vi "Interference 1065-366 Textfile.vi"() -> (3 "Tabelle für Textdatei":string[](array[string]))   [LabVIEW 2020, in "EPA 1065.lvlib" / "Interference verificaton 1065-366.lvlib"]
uses:
  Interference verificaton 1065-366.lvlib
  Visualisierungs Elemente/String - Ausgabefeld.ctl
  Ergebnis.ctl
  Sprachverwaltung/FGV Aktion Tabelle zerlegen.ctl
  Aktion FGV Interference.ctl
  Seiten/FT-IR/FGV FT-IR Aktionen.ctl
  Aktion Index uebersetzten.ctl
  Seiten/System Einstellungen V2/Aktioen FGV System Konstanten.ctl
  Sprachverwaltung/Sprachverwaltung.lvlib
  Seiten/System Einstellungen V2/System Einstellungen V2.lvlib
  Seiten/FT-IR/FT-IR.lvlib
panel:
  out "Tabellen-String":string
  out "Ergebnis":T1
  out "error out":errorcluster caption="Fehler (Ausgang)"
  in  "error in (no error)":errorcluster caption="Fehler (Eingang, kein Fehler)"
  out "max. Flow Weighted Mean:":T2 caption="%"
  out "Konzentration FlowWeightedMean":sgl=120.0 caption="Concentration:" min=0 format="%#.2f"
  out "Konzentration Komponente":sgl=120.0 caption="Concentration:" min=0
  out "Komponente:":T2 caption="ppm"
  out "[%]":sgl=120.0 caption="Interference:" min=0 format="%#.6g"
  out "Grenze in ppm:":sgl=2.0 min=0 format="%#.6g"
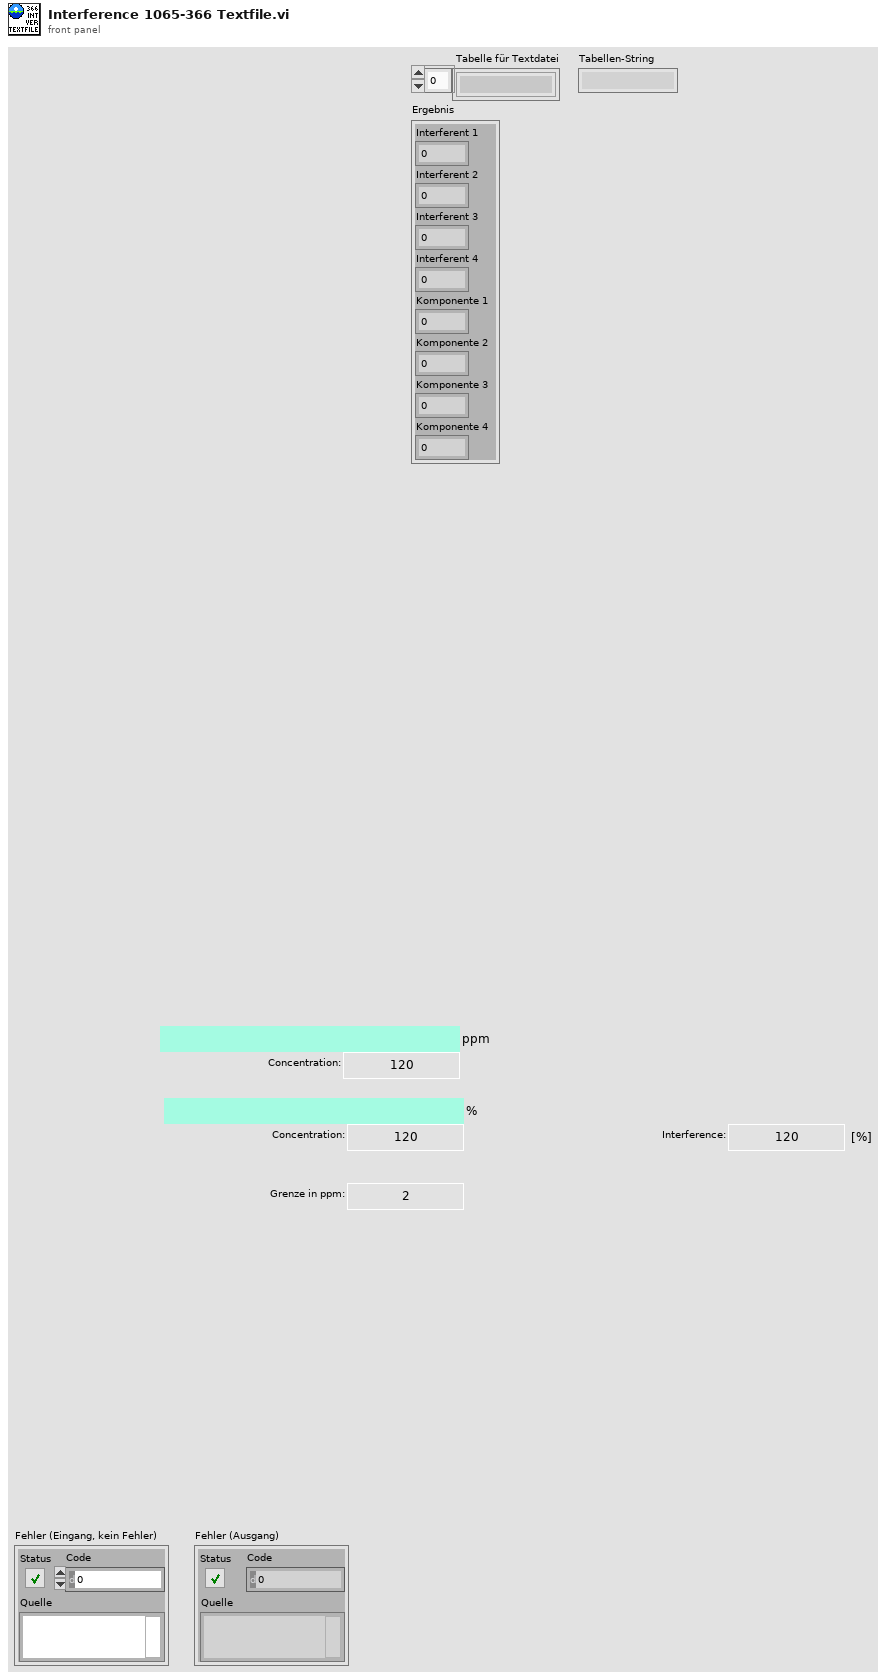
[diagram p1: front panel]
types:
  T1 = typedef "EPA 1065.lvlib/Interference verificaton 1065-366.lvlib/Ergebnis.ctl" = cluster{"Interferent 1":sgl, "Interferent 2":sgl, "Interferent 3":sgl, "Interferent 4":sgl, "Komponente 1":sgl, "Komponente 2":sgl, "Komponente 3":sgl, "Komponente 4":sgl}
  T2 = typedef "String - Ausgabefeld.ctl" = string
  T3 = typedef "System Einstellungen V2.lvlib/Aktioen FGV System Konstanten.ctl" = enum16{"lesen", "laden", "speichern", "Sprache"}
  T4 = typedef "EPA 1065.lvlib/Interference verificaton 1065-366.lvlib/Aktion Index uebersetzten.ctl" = enum16{"lesen", "schreiben", "auswerten"}
  T5 = typedef "FT-IR.lvlib/FGV FT-IR Aktionen.ctl" = enum16{"lesen", "NOG setzen", "NOS setzen", "Initialisieren", "speichern", "ALLES setzen", "FT-IR Spektrum loggen", "Komm Stoppen", "Spektrum LogKonfig"}
  T6 = typedef "EPA 1065.lvlib/Interference verificaton 1065-366.lvlib/Aktion FGV Interference.ctl" = enum16{"Lesen", "TestKonfig", "TestSetting", "Einheiten", "Ergebnis", "Laden", "Tabelle", "Speichern", "löschen"}
  T7 = typedef "Sprachverwaltung.lvlib/FGV Aktion Tabelle zerlegen.ctl" = enum16{"laden", "vereinzeln", "speichern"}
  T8 = typedef "EPA 1065.lvlib/Interference verificaton 1065-366.lvlib/TestSetting.ctl" = cluster{"Bearbeiter:":string, "Pfad:":path, "Textname:":string, "Analysator":T9}
  T9 = typedef "System Einstellungen V2.lvlib/Analysatoren.ctl" = string
  T10 = typedef "EPA 1065.lvlib/Interference verificaton 1065-366.lvlib/TestKonfig.ctl" = cluster{"CH4:":u16, "Ethane:":u16, "NMHC:":u16, "NMNEHC:":u16, "Komp 1 aktiv:":bool, "Komp 2 aktiv:":bool, "Komp 3 aktiv:":bool, "Komp 4 aktiv:":bool, "Modus":T11, "CG Aufschaltzeit:":dbl, "Interferent 1: CO2":u16, "Interferent 2: H2O":u16, "Interferent 3: CH4":u16, "Interferent 4: C2H6 / C3H8":u16, "Gasflaschen Nr.:":string, "Gasflaschen Nr.: 3":string, "Gasflaschen Nr.: 4":string, "Inter 1 aktiv":bool, "Inter 2 aktiv":bool, "Inter 3 aktiv":bool, "Inter 4 aktiv":bool, "Accuracy":string, "Accuracy 3":string, "Accuracy 4":string, "Konzentration 1:":dbl, "Konzentration 2:":dbl, "Konzentration 3:":dbl, "Konzentration 4:":dbl, "Flow weighted mean 1:":dbl, "Flow weighted mean 2:":dbl, "Flow weighted mean 3:":dbl, "Flow weighted mean 4:":dbl}
  T11 = typedef "EPA 1065.lvlib/Interference verificaton 1065-366.lvlib/Modus.ctl" = u16
  T12 = typedef "EPA 1065.lvlib/Interference verificaton 1065-366.lvlib/Komponenten.ctl" = cluster{"Komponente":T2, "Komponente Index":i32, "Komponente 2":T2, "Komponente Index 2":i32, "Komponente 3":T2, "Komponente Index 3":i32, "Komponente 4":T2, "Komponente Index 4":i32, "Interferent 1":T2, "Interferent Index":i32, "Interferent 2":T2, "Interferent 2 Index":i32, "Interferent 3":T2, "Interferent 3 Index":i32, "Interferent 4":T2, "Interferent 4 Index":i32}
  T13 = cluster{"Modell":string, "ProjektNummer":string, "Software Version":string, "Seriennummer":string}
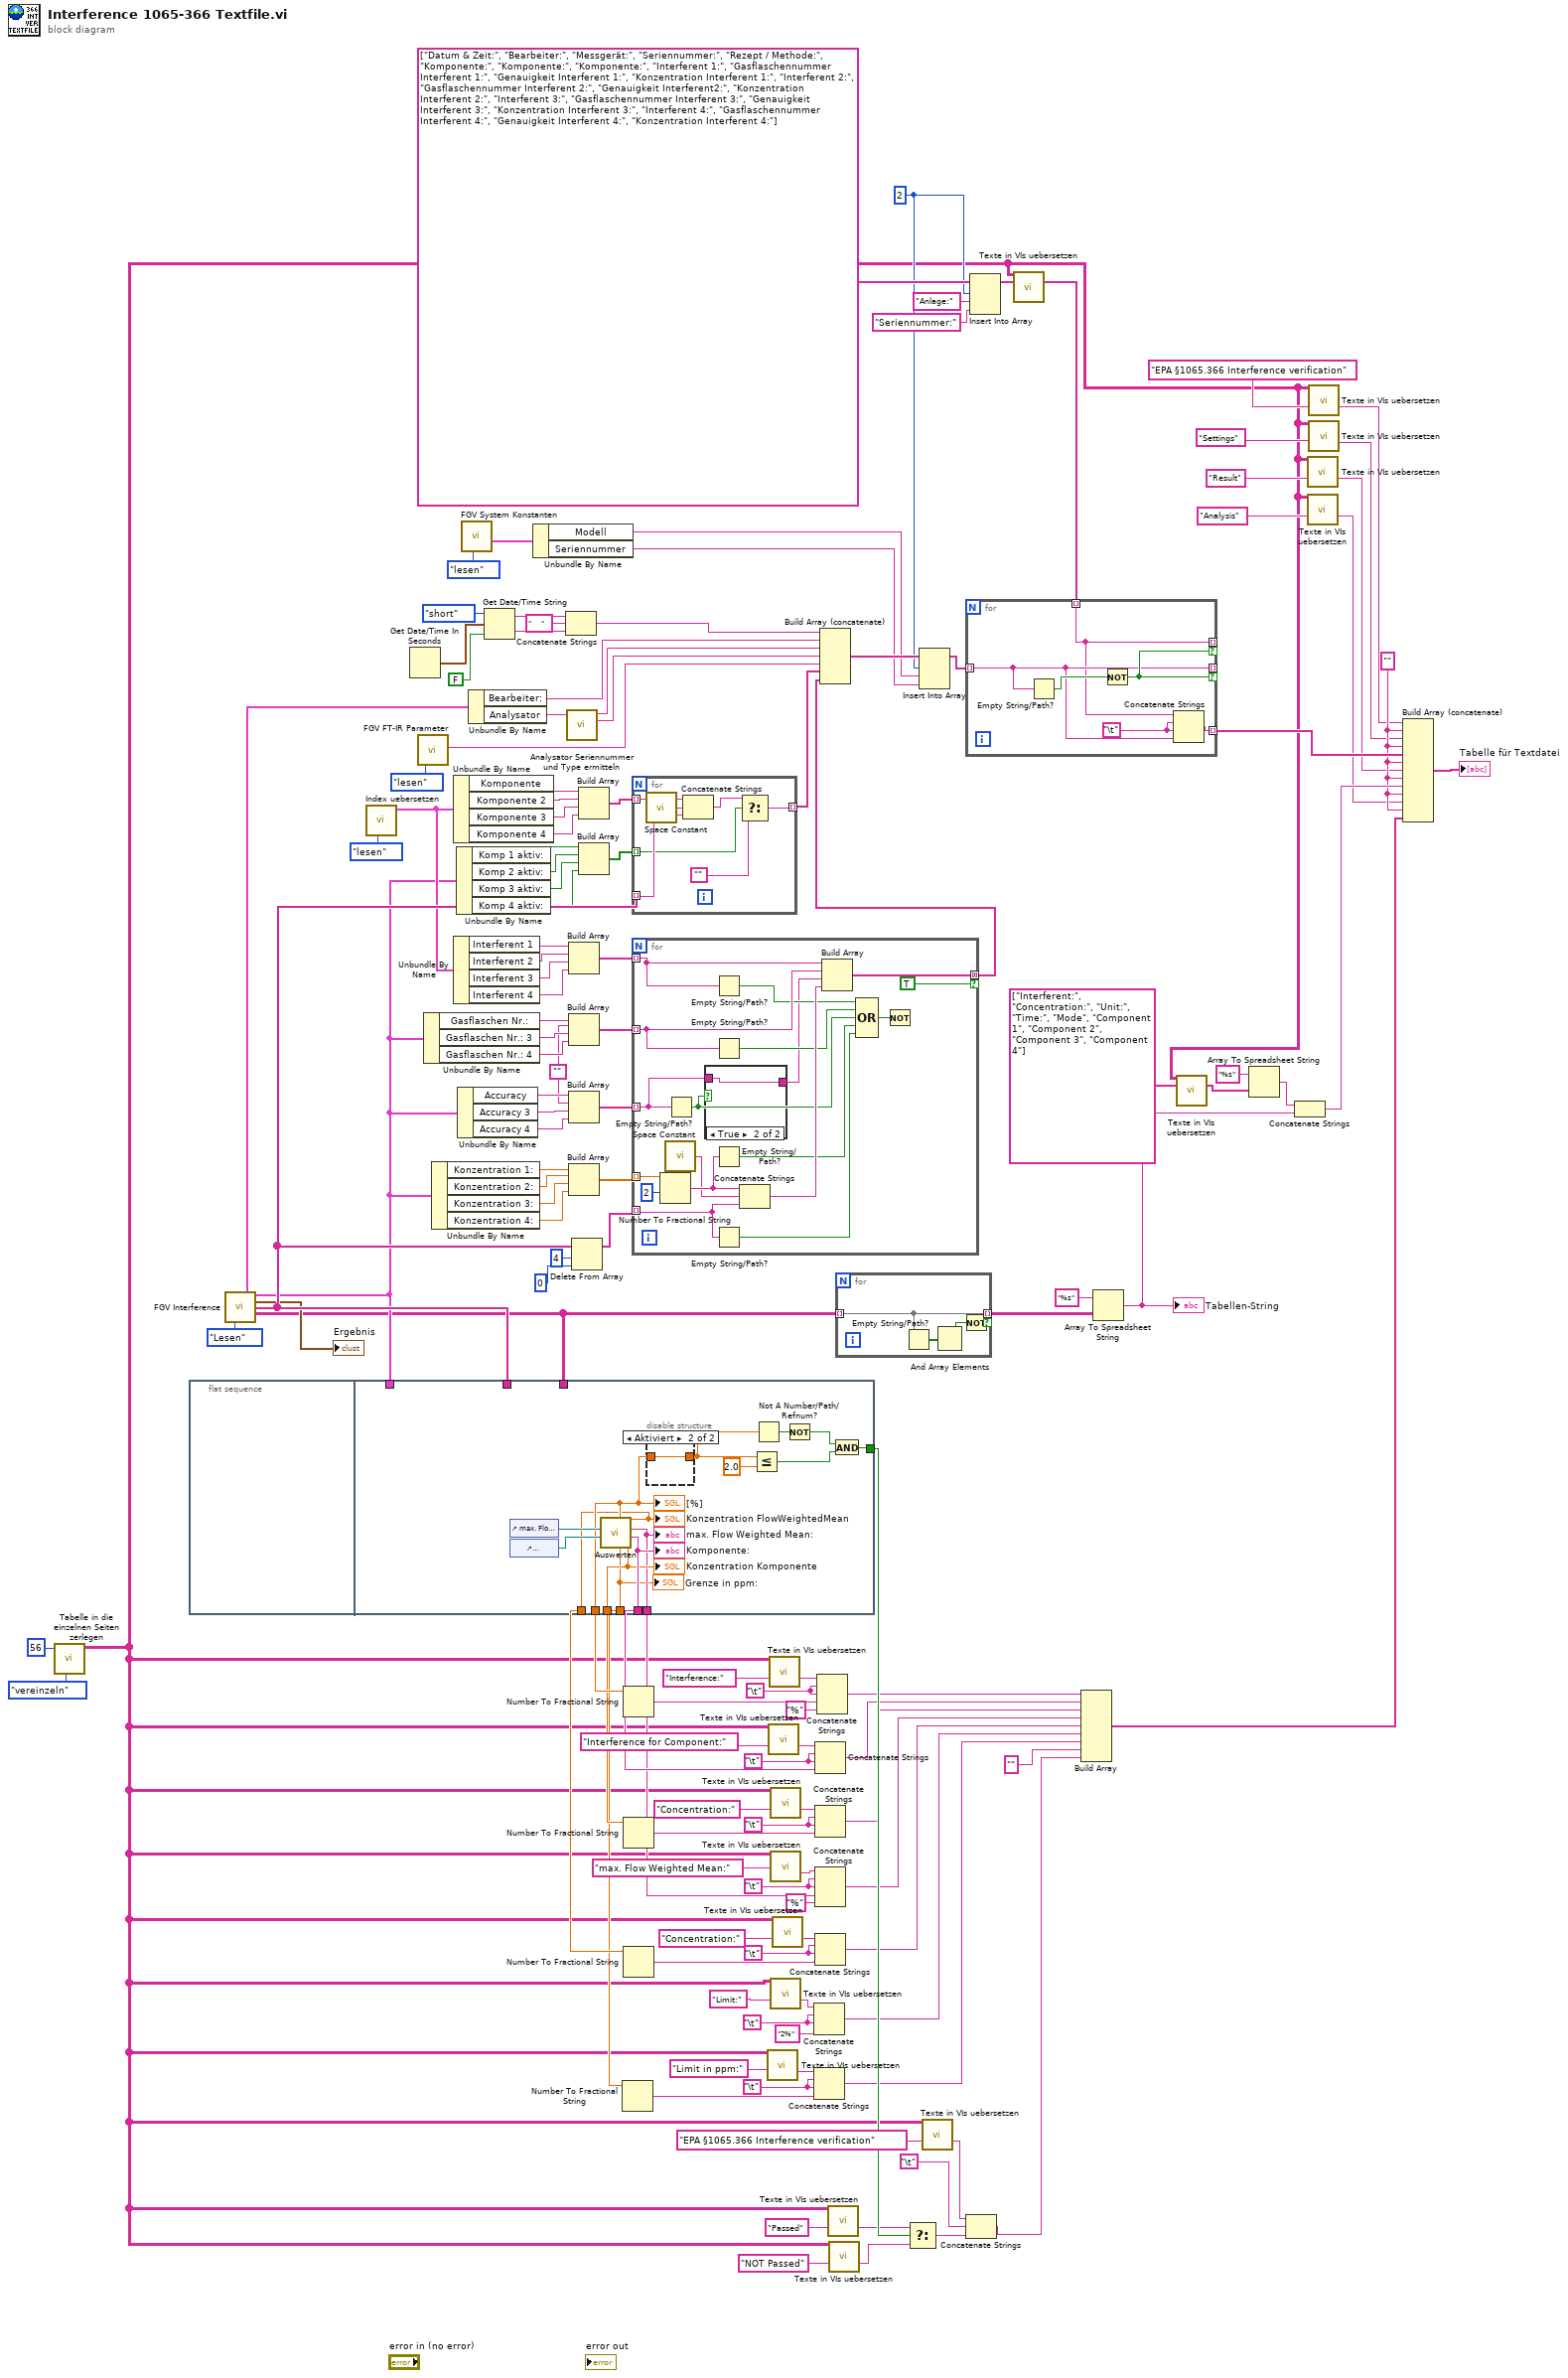
[diagram p0: block diagram]
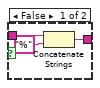
[diagram p2: hidden frame]
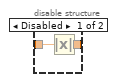
[diagram p3: hidden frame]
diagram:
  w40 = "" ("Element")
  w53 = "\t"
  w54 = "\t"
  w55 = "\t"
  w56 = "\t"
  w57 = "\t"
  w58 = "\t"
  w59 = "\t"
  w81 = ""
  w82 = 2 ("Index")
  n1 = call "Tabelle in die einzelnen Seiten zerlegen.vi"("Aktion"=FGV_Aktion_Tabelle_zerlegen."vereinzeln", "Index (Seite)"=56) -> ("Sprachliste"=w4:string[][])  [unwired: 7 in, 2 out]
  n2 = flat-sequence {
    tunnel: [w149] -> w140
    tunnel: w117 -> [_]
    tunnel: w45 -> [_]
    tunnel: w48 -> [_]
    tunnel: [w148] -> w79
    tunnel: [w147] -> w76
    tunnel: [w146] -> w72
    tunnel: [w145] -> w71
    tunnel: [w144] -> w66
    tunnel: [w143] -> w64
    frame #0 {
    }
    frame #1 {
      n3 = control-ref of="max. Flow Weighted Mean:"() -> (w156:refnum<vi>)
      n4 = control-ref of="Komponente:"() -> (w155:refnum<vi>)
      n5 = call "Auswerten.vi"("Komponente:"=w155, "max. Flow Weighted Mean:"=w156) -> ("Konzentration Komponente"=w146:dbl, "Komponente:"=w147:T2, "max. Flow Weighted Mean:"=w145:T2, "Konzentration FlowWeightedMean"=w144:dbl, "Limit in ppm"=w143:dbl, "[%]"=w148:dbl)  [unwired: 4 in]
      "max. Flow Weighted Mean:" <- w145
      "Konzentration FlowWeightedMean" <- w144
      "Konzentration Komponente" <- w146
      "Komponente:" <- w147
      "[%]" <- w148
      "Grenze in ppm:" <- w143
      n6 = disable-structure shown="Aktiviert" {
        disable-tunnel: [w158 w159] -> w153
        disable-tunnel: w148 -> [w157 w159]
        frame Disabled {
          n7 = Absolute Value(x=w157) -> (abs(x)=w158:dbl)
        }
        frame Enabled {
        }
      }
      n8 = Less Or Equal?(x=w153, y=2.0) -> (x <= y?=w151:bool)
      n9 = Not A Number/Path/Refnum?(number/path/refnum=w153) -> (NaN/Path/Refnum?=w152:bool)
      n10 = Not(x=w152) -> (.not. x?=w150:bool)
      n11 = And(x=w150, y=w151) -> (x .and. y?=w149:bool)
    }
  }
  n12 = call "FGV Interference.vi"("Aktion FGV Interference"=Aktion_FGV_Interference."Lesen") -> ("TestSetting"=w138:T8, "TestKonfig"=w48:T10, "Ergebnis"=→"Ergebnis":T1, "Êinheiten"=w117:string[], "Tabelle"=w45:T2[][])  [unwired: 9 in, 1 out]
  n13 = call "Index uebersetzen.vi"("Aktion"=Aktion_Index_uebersetzten."lesen") -> ("Komponenten"=w111:T12)  [unwired: 9 in, 1 out]
  n14 = Get Date/Time In Seconds() -> (seconds since 1Jan1904=w137:timestamp)
  n15 = call "FGV FT-IR Parameter.vi"("Aktion"=FGV_FT-IR_Aktionen."lesen") -> ("Current Recipe"=w118:string)  [unwired: 11 in, 7 out]
  n16 = Unbundle By Name(w48) -> ("Gasflaschen Nr.:"=w110:string, "Gasflaschen Nr.: 3"=w109:string, "Gasflaschen Nr.: 4"=w108:string)
  n17 = Unbundle By Name(w48) -> ("Konzentration 1:"=w107:dbl, "Konzentration 2:"=w106:dbl, "Konzentration 3:"=w105:dbl, "Konzentration 4:"=w104:dbl)
  n18 = Unbundle By Name(w111) -> ("Komponente"=w129:T2, "Komponente 2"=w128:T2, "Komponente 3"=w127:T2, "Komponente 4"=w38:T2)
  n19 = Unbundle By Name(w111) -> ("Interferent 1"=w115:T2, "Interferent 2"=w114:T2, "Interferent 3"=w113:T2, "Interferent 4"=w112:T2)
  n20 = Unbundle By Name(w48) -> ("Komp 1 aktiv:"=w126:bool, "Komp 2 aktiv:"=w125:bool, "Komp 3 aktiv:"=w124:bool, "Komp 4 aktiv:"=w37:bool)
  n21 = Unbundle By Name(w48) -> ("Accuracy"=w97:string, "Accuracy 3"=w96:string, "Accuracy 4"=w95:string)
  n22 = call "FGV System Konstanten.vi"("Aktionen"=Aktioen_FGV_System_Konstanten."lesen") -> ("Cluster out"=w90:T13)  [unwired: 6 in, 4 out]
  n23 = Unbundle By Name(w138) -> ("Bearbeiter:"=w120:string, "Analysator"=w3:T9)
  n24 = Get Date/Time String(date format (0)=enum16{"short", "long", "abbreviated"}."short" ("Datumsformat (0)"), seconds (now)=w137, want seconds? (F)=FALSE ("Angabe von Sekunden? (F)")) -> (date string=w136:string, time string=w135:string)
  n25 = Unbundle By Name(w90) -> ("Modell"=w86:string, "Seriennummer"=w85:string)
  n26 = Concatenate Strings(w136, "     " ("String"), w135) -> (w121:string)
  n27 = call "Analysator Seriennummer und Type ermitteln.vi"("Analysator"=w3) -> ("Type"=w2:string, "Name für Protokoll"=w1:string)  [unwired: 8 in, 1 out]
  n28 = Build Array(w115, w114, w113, w112) -> (w103:T2[])
  n29 = Build Array(w110, w81, w109, w108) -> (w102:string[])
  n30 = Build Array(w97, w81, w96, w95) -> (w94:string[])
  n31 = Build Array(w107, w106, w105, w104) -> (w101:dbl[])
  n32 = Delete From Array(array=w117, length=4 ("Länge"), index=0 ("Index")) -> (array with subset deleted=w99:string[])  [unwired: 1 out]
  n33 = Build Array(w129, w128, w127, w38) -> (w123:T2[])
  n34 = Build Array(w126, w125, w124, w37) -> (w122:bool[])
  n35 = Number To Fractional String(number=w64) -> (F-format string=w65:string)  [unwired: 3 in]
  n36 = Number To Fractional String(number=w79) -> (F-format string=w80:string)  [unwired: 3 in]
  n37 = Number To Fractional String(number=w72) -> (F-format string=w73:string)  [unwired: 3 in]
  n38 = Number To Fractional String(number=w66) -> (F-format string=w67:string)  [unwired: 3 in]
  n39 = for {
    tunnel: [w163] -> w119 mode=indexing
    tunnel: w123 -> [w166] mode=indexing
    tunnel: w122 -> [w162] mode=indexing
    tunnel: w117 -> [w165] mode=indexing
    n40 = call <vilib>:"Space Constant.vi"() -> ("String"=w164:string)
    n41 = Concatenate Strings(w166, w164, w165) -> (w161:string)
    n42 = Select(t=w161, s=w162, f="") -> (s? t:f=w163:string)
  }
  n43 = for {
    tunnel: w103 -> [w181] mode=indexing
    tunnel: w102 -> [w180] mode=indexing
    tunnel: w101 -> [w184] mode=indexing
    tunnel: w99 -> [w183] mode=indexing
    tunnel: [w178] -> w98 mode=concatenating if=TRUE
    tunnel: w94 -> [w168] mode=indexing
    n44 = Number To Fractional String(number=w184, precision (6)=i16 2 ("Genauigkeit (6)")) -> (F-format string=w182:string)  [unwired: 2 in]
    n45 = call <vilib>:"Space Constant.vi"() -> ("String"=w172:string)
    n46 = Empty String/Path?(string/path=w168) -> (empty?=w167:bool)
    n47 = case shown="True" w167 {
      tunnel: [w186 w188] -> w171
      tunnel: w168 -> [w185 w188]
      frame False {
        n48 = Concatenate Strings(w185, "%" ("String")) -> (w186:string)
      }
      frame True {
      }
    }
    n49 = Empty String/Path?(string/path=w181) -> (empty?=w177:bool)
    n50 = Empty String/Path?(string/path=w180) -> (empty?=w176:bool)
    n51 = Empty String/Path?(string/path=w182) -> (empty?=w173:bool)
    n52 = Empty String/Path?(string/path=w183) -> (empty?=w175:bool)
    n53 = Concatenate Strings(w182, w172, w183) -> (w179:string)
    n54 = Build Array(w181, w180, w171, w179) -> (w178:T2[])
    n55 = Compound Arithmetic op=OR ("Mehrfacharithmetik")(w177, w176, w167, w173, w175) -> (w174:bool)
    n56 = Not(x=w174) -> ()  [unwired: 1 out]
  }
  n57 = call "Texte in VIs uebersetzen.vi"("Sprachliste"=w4, "String zum Übersetzen"="Limit in ppm:" ("String")) -> ("String zum Übersetzen"=w13:string)  [unwired: 9 in, 4 out]
  n58 = call "Texte in VIs uebersetzen.vi"("Sprachliste"=w4, "String zum Übersetzen"="Interference for Component:" ("String")) -> ("String zum Übersetzen"=w23:string)  [unwired: 9 in, 4 out]
  n59 = call "Texte in VIs uebersetzen.vi"("Sprachliste"=w4, "String zum Übersetzen"="Interference:" ("String")) -> ("String zum Übersetzen"=w25:string)  [unwired: 9 in, 4 out]
  n60 = call "Texte in VIs uebersetzen.vi"("Sprachliste"=w4, "String zum Übersetzen"="Concentration:" ("String")) -> ("String zum Übersetzen"=w22:string)  [unwired: 9 in, 4 out]
  n61 = call "Texte in VIs uebersetzen.vi"("Sprachliste"=w4, "String zum Übersetzen"="max. Flow Weighted Mean:" ("String")) -> ("String zum Übersetzen"=w20:string)  [unwired: 9 in, 4 out]
  n62 = call "Texte in VIs uebersetzen.vi"("Sprachliste"=w4, "String zum Übersetzen"="Limit:" ("String")) -> ("String zum Übersetzen"=w16:string)  [unwired: 9 in, 4 out]
  n63 = call "Texte in VIs uebersetzen.vi"("Sprachliste"=w4, "String zum Übersetzen"="Concentration:" ("String")) -> ("String zum Übersetzen"=w18:string)  [unwired: 9 in, 4 out]
  n64 = Concatenate Strings(w16, w53, w53, "2%" ("String")) -> (w51:string)
  n65 = Concatenate Strings(w13, w54, w54, w65) -> (w52:string)
  n66 = Concatenate Strings(w23, w58, w58, w76) -> (w75:string)
  n67 = Concatenate Strings(w22, w57, w57, w73) -> (w74:string)
  n68 = Concatenate Strings(w20, w56, w56, w71, T2 "%" ("String")) -> (w70:string)
  n69 = Concatenate Strings(w18, w55, w55, w67) -> (w68:string)
  n70 = Concatenate Strings(w25, w59, w59, w80, "%" ("String")) -> (w77:string)
  n71 = Build Array (concatenate)(w121, w120, w1, w2, w118, w119, w98) -> (w88:T2[])
  n72 = call "Texte in VIs uebersetzen.vi"("Sprachliste"=w4, "String zum Übersetzen"=T2 "Passed" ("String")) -> ("String zum Übersetzen"=w9:string)  [unwired: 9 in, 4 out]
  n73 = call "Texte in VIs uebersetzen.vi"("Sprachliste"=w4, "String zum Übersetzen"=T2 "NOT Passed" ("String")) -> ("String zum Übersetzen"=w7:string)  [unwired: 9 in, 4 out]
  n74 = for {
    tunnel: w45 -> [w192] mode=indexing
    tunnel: [w192] -> w44 mode=indexing if=w189
    n75 = Empty String/Path?(string/path=w192) -> (empty?=w191:bool[])
    n76 = And Array Elements(Boolean array=w191) -> (logical AND=w190:bool)
    n77 = Not(x=w190) -> (.not. x?=w189:bool)
  }
  n78 = Select(t=w9, s=w140, f=w7) -> (s? t:f=w11:string)
  n79 = Insert Into Array(array=w88, index=w82, new element #1=w86, new element #2=w85) -> (w87:T2[])
  n80 = call "Texte in VIs uebersetzen.vi"("Sprachliste"=w4, "String zum Übersetzen"="EPA §1065.366 Interference verification") -> ("String zum Übersetzen"=w5:string)  [unwired: 9 in, 4 out]
  n81 = Concatenate Strings(w5, "\t", w11) -> (w12:string)
  n82 = Insert Into Array(array=string[] ["Datum & Zeit:", "Bearbeiter:", "Messgerät:", "Seriennummer:", "Rezept / Methode:", "Komponente:", "Komponente:", "Komponente:", "Interferent 1:", "Gasflaschennummer Interferent 1:", "Genauigkeit Interferent 1:", "Konzentration Interferent 1:", "Interferent 2:", "Gasflaschennummer Interferent 2:", "Genauigkeit Interferent2:", "Konzentration Interferent 2:", "Interferent 3:", "Gasflaschennummer Interferent 3:", "Genauigkeit Interferent 3:", "Konzentration Interferent 3:", "Interferent 4:", "Gasflaschennummer Interferent 4:", "Genauigkeit Interferent 4:", "Konzentration Interferent 4:"], index=w82, new element #1="Anlage:" ("Neues Element/Teil-Array"), new element #2="Seriennummer:" ("Neues Element/Teil-Array")) -> (w89:string[])
  n83 = call "Texte in VIs uebersetzen.vi"("Sprachliste"=w4, "String-Array zum Übersetzen"=w89) -> ("String-Array zum Übersetzen"=w92:string[])  [unwired: 9 in, 4 out]
  n84 = for {
    tunnel: w87 -> [w196] mode=indexing
    tunnel: [w196] -> _ mode=indexing if=w197
    tunnel: [w194] -> _ mode=indexing if=w197
    tunnel: w92 -> [w194] mode=indexing
    tunnel: [w195] -> w62 mode=indexing
    w193 = "\t"
    n85 = Empty String/Path?(string/path=w196) -> (empty?=w198:bool)
    n86 = Not(x=w198) -> (.not. x?=w197:bool)
    n87 = Concatenate Strings(w194, w193, w193, w196) -> (w195:string)
  }
  n88 = Build Array(w77, w75, w74, w70, w68, w51, w52, "" ("Element"), w12) -> (w61:string[])
  n89 = Array To Spreadsheet String(array=w44, 3:"%s" ("Format-String")) -> (spreadsheet string=w42:string)  [unwired: 1 in]
  "Tabellen-String" <- w42
  n90 = call "Texte in VIs uebersetzen.vi"("Sprachliste"=w4, "String-Array zum Übersetzen"=string[] ["Interferent:", "Concentration:", "Unit:", "Time:", "Mode", "Component 1", "Component 2", "Component 3", "Component 4"]) -> ("String-Array zum Übersetzen"=w27:string[])  [unwired: 9 in, 4 out]
  n91 = Array To Spreadsheet String(array=w27, 3:"%s" ("Format-String")) -> (spreadsheet string=w43:string)  [unwired: 1 in]
  n92 = Concatenate Strings(w43, w42) -> (w41:string)
  n93 = call "Texte in VIs uebersetzen.vi"("Sprachliste"=w4, "String zum Übersetzen"="Result" ("Element")) -> ("String zum Übersetzen"=w31:string)  [unwired: 9 in, 4 out]
  n94 = call "Texte in VIs uebersetzen.vi"("Sprachliste"=w4, "String zum Übersetzen"="Analysis" ("Element")) -> ("String zum Übersetzen"=w30:string)  [unwired: 9 in, 4 out]
  n95 = call "Texte in VIs uebersetzen.vi"("Sprachliste"=w4, "String zum Übersetzen"="EPA §1065.366 Interference verification" ("Element")) -> ("String zum Übersetzen"=w35:string)  [unwired: 9 in, 4 out]
  n96 = call "Texte in VIs uebersetzen.vi"("Sprachliste"=w4, "String zum Übersetzen"="Settings" ("Element")) -> ("String zum Übersetzen"=w33:string)  [unwired: 9 in, 4 out]
  n97 = Build Array (concatenate)(w35, w40, w33, w40, w62, w40, w31, w40, w41, w40, w30, w40, w61) -> (→"Tabelle für Textdatei":string[])
